vi "Configure Trigger.vi"(0 "Instrument handles in":refnum<k15>[](array[refnum]), 5 "Channels Name":string[](array[string]), 7 "Relative To":T1[](array[typedef]) items=["Power sequence start", "Previous source start", "Previous source end"], 11 "error in (no error)":errorcluster) -> (15 "error out":errorcluster)   [LabVIEW 2024, in "devicePowerSequencerCoreLogic.lvlib"]
uses:
  devicePowerSequencerCoreLogic.lvlib
  controls/Relative To.ctl
  <instrlib>/niDCPower/nidcpower.llb/niDCPower Digital Edge - Edge.ctl
  <instrlib>/niDCPower/nidcpower.llb/niDCPower Disable Start Trigger With Channels.vi
  <instrlib>/niDCPower/nidcpower.llb/niDCPower Configure Digital Edge Start Trigger With Channels.vi
  Device Power Sequencer.lvlib
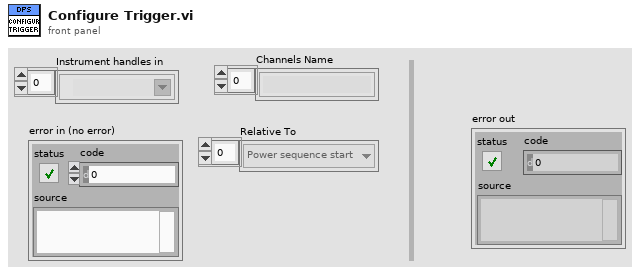
[diagram p1: front panel]
types:
  T1 = typedef "Device Power Sequencer.lvlib/Relative To.ctl" = u32
  T2 = typedef "niDCPower Digital Edge - Edge.ctl" = i32
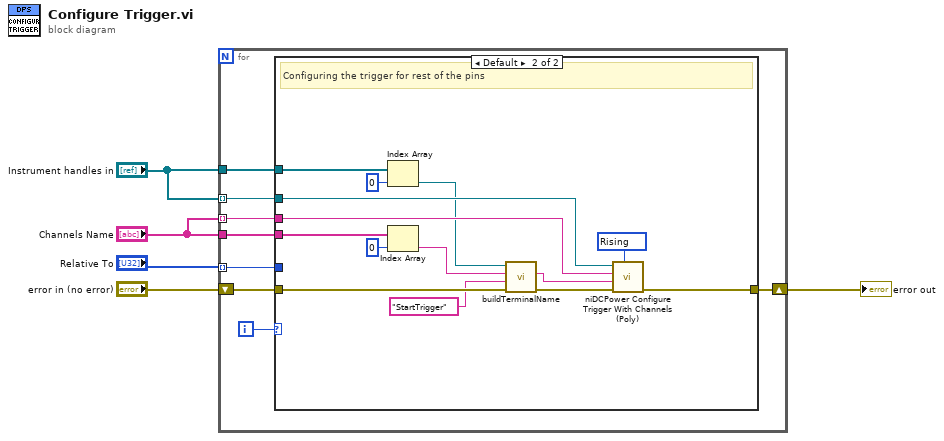
[diagram p0: block diagram]
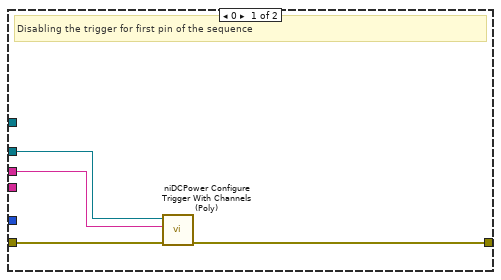
[diagram p2: hidden frame]
diagram:
  n1 = for {
    tunnel: "Instrument handles in" -> [w8] mode=indexing
    shift-right: [w11] -> w3
    shift-left: "error in (no error)" -> [w12]
    tunnel: "Relative To" -> [w10] mode=indexing
    tunnel: "Channels Name" -> [w9]
    tunnel: "Channels Name" -> [w7] mode=indexing
    tunnel: "Instrument handles in" -> [w6]
    i -> [w13]
    n2 = case shown="Default" w13 {
      tunnel: w12 -> [w17 w31]
      tunnel: [w16 w30] -> w11
      tunnel: w10 -> [_ _]
      tunnel: w9 -> [_ w29]
      tunnel: w8 -> [w15 w28]
      tunnel: w7 -> [w14 w27]
      tunnel: w6 -> [_ w26]
      frame 0 {
        # "Disabling the trigger for first pin of the sequence"
        n3 = call-poly <instrlib>:"niDCPower Configure Trigger With Channels (Poly).vi"("error in (no error)"=w17, "channel name"=w14, "instrument handle"=w15) -> ("error out"=w16:errorcluster)  [unwired: 7 in, 1 out]
      }
      frame Default {
        w23 = T2 1016 items=["Rising"=1016, "Falling"=1017] ("edge (rising)")
        # "Configuring the trigger for rest of the pins"
        n4 = Index Array(array=w26, index=0) -> (element=w22:refnum<k15>)
        n5 = Index Array(array=w29, index=0) -> (element=w21:string)
        n6 = call "buildTerminalName.vi"("error in (no error)"=w31, "Local Terminal Name"="StartTrigger", "Channel Name"=w21, "session handle"=w22) -> ("error IO"=w19:errorcluster, "Fully Qualified Terminal Name"=w18:string)  [unwired: 5 in, 1 out]
        n7 = call-poly <instrlib>:"niDCPower Configure Trigger With Channels (Poly).vi"("edge (rising)"=w23, "error in (no error)"=w19, "input terminal"=w18, "channel name"=w27, "instrument handle"=w28) -> ("error out"=w30:errorcluster)  [unwired: 5 in, 1 out]
      }
    }
  }
  "error out" <- w3
